vi "Switch Open Close.vi"(6 "Measurement":T1, 7 "Open/Close (F: Open)":bool, 8 "error in (no error)":errorcluster, 11 "VISA resource name in":refnum<visa-resource-name>) -> (0 "error out":errorcluster, 3 "VISA resource name out":refnum<visa-resource-name>)   [LabVIEW 2016, in "Hall Effect Library.lvlib"]
uses:
  Hall Effect Library.lvlib
  Controls/Measurement.ctl
  Global Variables/Instruments.vi
  Global Variables/Test Settings.vi
  Switch Open Close (3706).vi
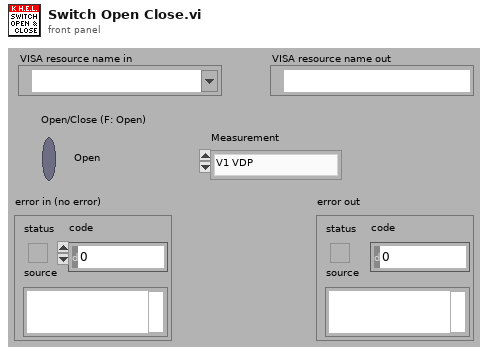
[diagram p1: front panel]
types:
  T1 = typedef "Hall Effect Library.lvlib/Measurement.ctl" = enum16{"V1 VDP", "V2 VDP", "V3 VDP", "V4 VDP", "V5 VDP", "V6 VDP", "V7 VDP", "V8 VDP", "V1 HE", "V2 HE", "V3 HE", "V4 HE", "V5 HE", "V6 HE", "V7 HE", "V8 HE", "V1 Res Bar", "V1 Hall Bar", "V1 Res 6-Cot", "V2 Res 6-Cot", "V3 Res 6-Cot", "V4 Res 6-Cot", "V1 Hall 6-Cot", "V2 Hall 6-Cot", "V3 Hall 6-Cot", "V4 Hall 6-Cot", "V5 Hall 6-Cot", "V6 Hall 6-Cot", "V7 Hall 6-Cot", "V8 Hall 6-Cot", "V1 Res 8-Cot", "V2 Res 8-Cot", "V3 Res 8-Cot", "V4 Res 8-Cot", "V1 Hall 8-Cot", "V2 Hall 8-Cot", "V3 Hall 8-Cot", "V4 Hall 8-Cot"}
  T2 = typedef "Hall Effect Library.lvlib/Switches.ctl" = enum16{"3706A"}
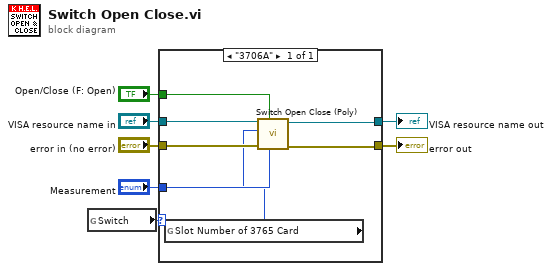
[diagram p0: block diagram]
diagram:
  n1 = global read "Instruments.vi" "Switch"() -> (w7:T2)
  n2 = case shown="\"3706A\"" w7 {
    tunnel: "VISA resource name in" -> [w14]
    tunnel: "error in (no error)" -> [w13]
    tunnel: [w11] -> w2
    tunnel: [w12] -> w1
    tunnel: "Measurement" -> [w9]
    tunnel: "Open/Close (F: Open)" -> [w10]
    frame "3706A" {
      n3 = global read "Test Settings.vi" "Slot Number of 3765 Card"() -> (w8:u32)
      n4 = call-poly "Switch Open Close (Poly).vi"("Measurement"=w9, "Open/Close (F: Open)"=w10, "error in (no error)"=w13, "Slot Number"=w8, "VISA resource name in"=w14) -> ("error out"=w11:errorcluster, "VISA resource name out"=w12:refnum<visa-resource-name>)  [unwired: 5 in]
    }
  }
  "error out" <- w2
  "VISA resource name out" <- w1
